vi "find humidity.vi"(11 "Array in":sgl[](array[numeric])) -> (3 "Array out":sgl[](array[numeric]))   [LabVIEW 2020, in "Sensor910.lvclass"]
uses:
  Sensor910.lvclass
  Sensor910.lvclass/Sensor910.ctl
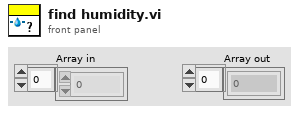
[diagram p1: front panel]
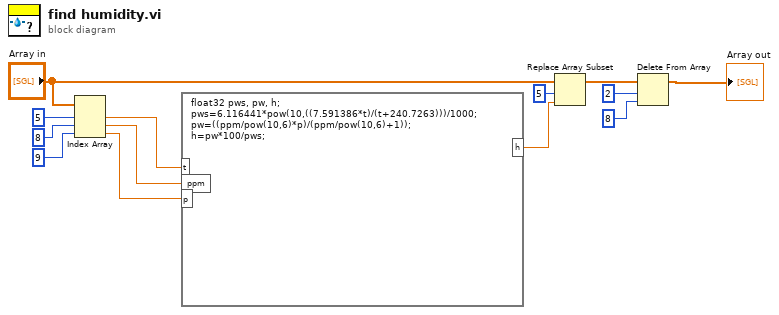
[diagram p0: block diagram]
diagram:
  n1 = Index Array(array="Array in", index #1=5 ("index"), index #2=8 ("index"), index #3=9 ("index")) -> (element #1=w10:sgl, element #2=w9:sgl, element #3=w8:sgl)
  n2 = formula code="float32 pws, pw, h;\npws=6.116441*pow(10,((7.591386*t)/(t+240.7263)))/1000;\npw=((ppm/pow(10,6)*p)/(ppm/pow(10,6)+1));\nh=pw*100/pws;"("t"=w10, "ppm"=w9, "p"=w8) -> ("h"=w5:sgl)
  n3 = Replace Array Subset(array="Array in", new element=w5, index=5) -> (w4:sgl[])
  n4 = Delete From Array(array=w4, length=2, index=8) -> (array with subset deleted=→"Array out":sgl[])  [unwired: 1 out]
